vi "PythonProcessNameIndex.vi"(8 "OP":enum16{"Init", "Get"}(ring)=enum."Get", 11 "PythonNode":string) -> (3 "PythonTCP/IP":refnum<k5>, 4 "PythonProcessNameList":string[](array[string]))   [LabVIEW 2020]
uses:
  <vilib>/Utility/error.llb/DialogType.ctl
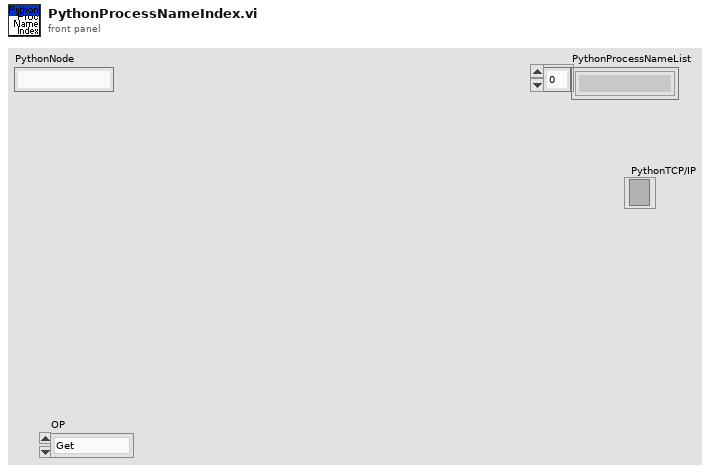
[diagram p1: front panel]
types:
  T1 = typedef "DialogType.ctl" = u16
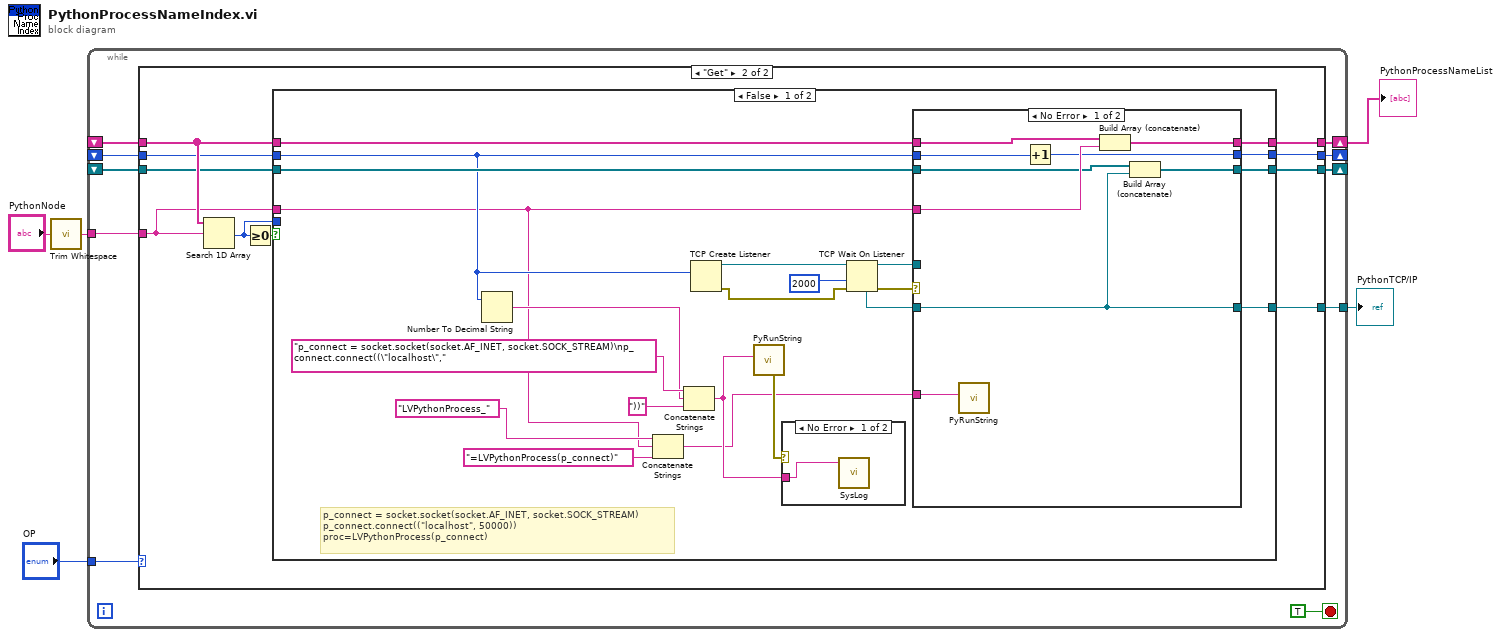
[diagram p0: block diagram]
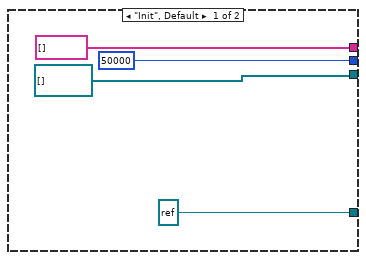
[diagram p2: hidden frame]
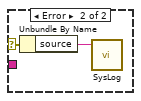
[diagram p3: hidden frame]
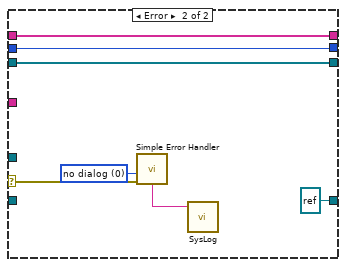
[diagram p4: hidden frame]
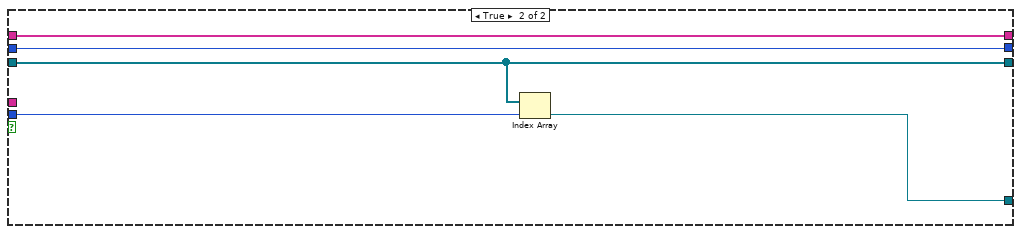
[diagram p5: hidden frame]
diagram:
  n1 = call <vilib>:"Trim Whitespace.vi"("string"="PythonNode") -> ("trimmed string"=w4:string)  [unwired: 1 in]
  n2 = while {
    tunnel: "OP" -> [w14]
    tunnel: w4 -> [w13]
    shift-right: [w12] -> w1
    shift-left: _ -> [w11]
    shift-right: [w10] -> _
    shift-left: _ -> [w9]
    shift-right: [w8] -> _
    shift-left: _ -> [w7]
    tunnel: [w6] -> w2
    stop <- TRUE stop-if-true
    n3 = case shown="\"Get\"" w14 {
      tunnel: w13 -> [_ w26]
      tunnel: [string[] [] w25] -> w12
      tunnel: w11 -> [_ w28]
      tunnel: [u16 50000 ("port") w24] -> w10
      tunnel: w9 -> [_ w27]
      tunnel: [refnum<k5>[] [] w23] -> w8
      tunnel: w7 -> [_ w22]
      tunnel: [refnum<k5> refnum ("listener ID") w21] -> w6
      frame "Init", Default {
      }
      frame "Get" {
        n4 = Search 1D Array(1D array=w28, element=w26) -> (index of element=w20:i32)  [unwired: 1 in]
        n5 = Greater Or Equal To 0?(x=w20) -> (x >= 0?=w29:bool)
        n6 = case shown="False" w29 {
          tunnel: w28 -> [w49 w75]
          tunnel: w27 -> [w42 w74]
          tunnel: w26 -> [w33 _]
          tunnel: [w48 w75] -> w25
          tunnel: [w47 w74] -> w24
          tunnel: [w45 w72] -> w23
          tunnel: w22 -> [w44 w72]
          tunnel: [w43 w71] -> w21
          tunnel: w20 -> [_ w73]
          frame False {
            # "p_connect = socket.socket(socket.AF_INET, socket.SOCK_STREAM)\np_connect.connect((\"localhost\", 50000))\nproc=LVPythonProcess(p_connect)"
            n7 = Number To Decimal String(number=w42) -> (decimal integer string=w38:string)  [unwired: 1 in]
            n8 = Concatenate Strings("LVPythonProcess_" ("string"), w33, "=LVPythonProcess(p_connect)" ("string")) -> (w30:string)
            n9 = Concatenate Strings("p_connect = socket.socket(socket.AF_INET, socket.SOCK_STREAM)\np_connect.connect((\"localhost\"," ("string"), w38, "))" ("string")) -> (w40:string)
            n10 = TCP Create Listener(10:w42) -> (0:w32:errorcluster, 3:w51:refnum<k5>)  [unwired: 4 in, 1 out]
            n11 = call "PyRunString.vi"("PyScript"=w40) -> ("Python Err"=w41:errorcluster)  [unwired: 9 in, 1 out]
            n12 = case shown="No Error" w41 {
              selector: w41 -> [_ w54]
              tunnel: w40 -> [w52 _]
              frame No Error {
                n13 = call "SysLog.vi"("Mssage"=w52) -> ()  [unwired: 5 in]
              }
              frame Error {
                n14 = Unbundle By Name(w54) -> ("source"=w53:string)
                n15 = call "SysLog.vi"("Mssage"=w53) -> ()  [unwired: 5 in]
              }
            }
            n16 = TCP Wait On Listener(8:w32, 9:2000 ("timeout ms (wait forever: -1)"), 11:w51) -> (0:w31:errorcluster, 3:w36:refnum<k5>, 4:w46:refnum<k5>)  [unwired: 1 in, 2 out]
            n17 = case shown="No Error" w31 {
              selector: w31 -> [_ w66]
              tunnel: w33 -> [w62 _]
              tunnel: w49 -> [w63 w70]
              tunnel: [w61 w70] -> w48
              tunnel: w42 -> [w60 w69]
              tunnel: [w59 w69] -> w47
              tunnel: w46 -> [w56 _]
              tunnel: [w58 w68] -> w45
              tunnel: w44 -> [w57 w68]
              tunnel: [w56 refnum<k5> refnum ("listener ID")] -> w43
              tunnel: w36 -> [_ _]
              tunnel: w30 -> [w55 _]
              frame No Error {
                n18 = call "PyRunString.vi"("PyScript"=w55) -> ()  [unwired: 9 in, 2 out]
                n19 = Increment(x=w60) -> (x+1=w59:u16)
                n20 = Build Array (concatenate)(w63, w62) -> (w61:string[])
                n21 = Build Array (concatenate)(w57, w56) -> (w58:refnum<k5>[])
              }
              frame Error {
                w65 = T1 0 items=["no dialog", "OK message", "continue or stop message", "OK message + warnings", "continue/stop + warnings"] ("type of dialog (OK msg:1)")
                n22 = call <vilib>:"Simple Error Handler.vi"("type of dialog (OK msg:1)"=w65, "error in (no error)"=w66) -> ("message"=w64:string)  [unwired: 3 in, 4 out]
                n23 = call "SysLog.vi"("Mssage"=w64) -> ()  [unwired: 5 in]
              }
            }
          }
          frame True {
            n24 = Index Array(array=w72, index=w73) -> (element=w71:refnum<k5>)
          }
        }
      }
    }
  }
  "PythonTCP/IP" <- w2
  "PythonProcessNameList" <- w1
